vi "Write Test Executive Ref.vi"(10 "Test Executive Ref":refnum<data-value>, 11 "Test Executive Builder Model in":refnum<class "Test Executive Builder Model.lvclass">) -> (3 "Test Executive Builder Model out":refnum<class "Test Executive Builder Model.lvclass">)   [LabVIEW 2017, in "Test Executive Builder Model.lvclass"]
uses:
  Test Executive Builder Model.lvclass
  <vilib>/gpm_packages/@cs/test-executive/Source/Test Executive/ITestExecutive/ITest Executive.lvclass
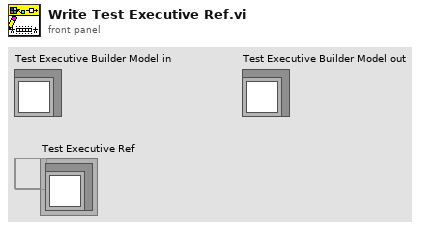
[diagram p1: front panel]
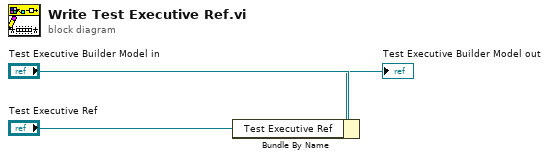
[diagram p0: block diagram]
diagram:
  n1 = Bundle By Name(cluster="Test Executive Builder Model in", "Test Executive Ref"="Test Executive Ref") -> (→"Test Executive Builder Model out":refnum<class "Test Executive Builder Model.lvclass">)
